vi "GEOM_GetCmdLineArgs.vi"() -> (6 "det_database":path, 8 "port":u16=4080, 13 "exit":bool, 14 "fpa":string)   [LabVIEW 2016]
panel:
  out "error out":errorcluster
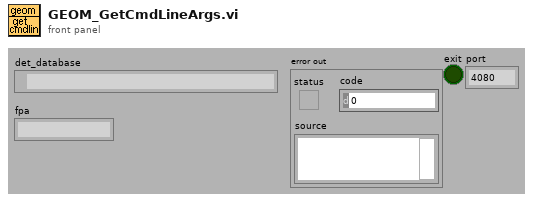
[diagram p1: front panel]
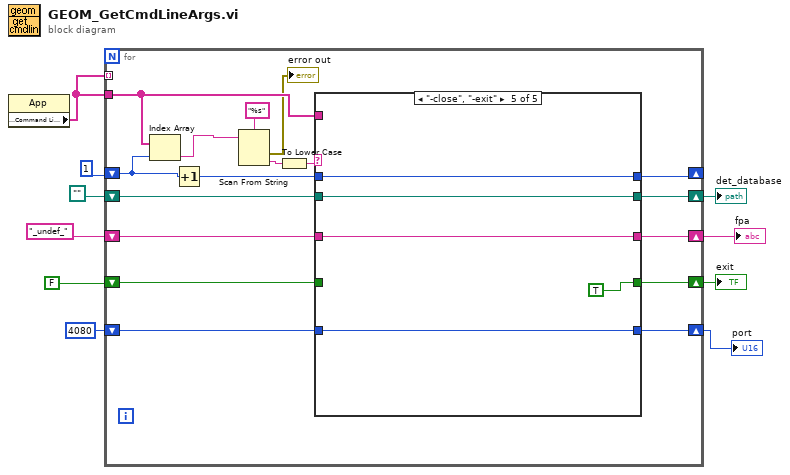
[diagram p0: block diagram]
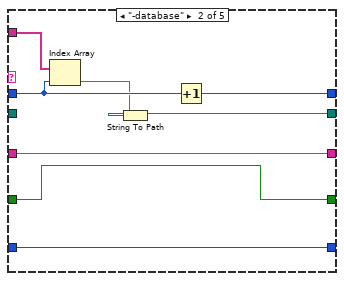
[diagram p3: hidden frame]
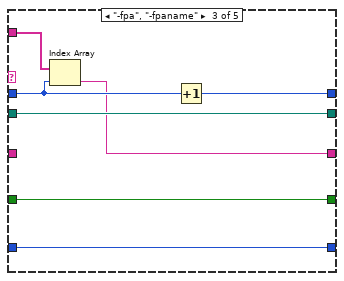
[diagram p4: hidden frame]
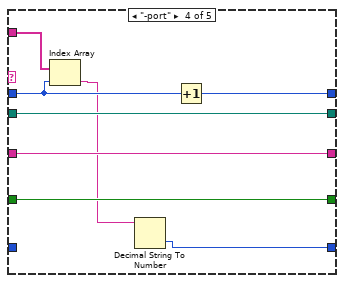
[diagram p5: hidden frame]
diagram:
  n1 = property class="App"() -> ("Application:Command Line Arguments"=w7:string[])  [unwired: 2 in, 2 out]
  n2 = for {
    shift-right: [w27] -> w9
    shift-left: path "" -> [w26]
    tunnel: w7 -> [w23]
    shift-right: [w21] -> _
    shift-left: 1 ("index") -> [w24]
    tunnel: w7 -> [_] mode=indexing
    shift-right: [w15] -> w6
    shift-left: "_undef_" ("element") -> [w16]
    shift-right: [w13] -> w3
    shift-left: FALSE -> [w14]
    shift-right: [w12] -> w2
    shift-left: 4080 -> [w11]
    n3 = Index Array(array=w23, index=w24) -> (element=w22:string)
    n4 = Increment(x=w24) -> (x+1=w25:i32)
    n5 = Scan From String(format string="%s", input string=w22) -> (error out=→"error out":errorcluster, output 1=w18:string)  [unwired: 2 in, 3 out]
    n6 = To Lower Case(string=w18) -> (all lower case string=w19:string)
    n7 = case shown="\"-close\", \"-exit\"" w19 {
      tunnel: [w32 w40 w44 w52 w59] -> w27
      tunnel: w26 -> [w32 _ w44 w52 w59]
      tunnel: w23 -> [_ w39 w47 w55 _]
      tunnel: w25 -> [w31 w38 w46 w54 w60]
      tunnel: [w31 w37 w45 w53 w60] -> w21
      tunnel: w16 -> [w30 w36 _ w50 w58]
      tunnel: [w30 w36 w43 w50 w58] -> w15
      tunnel: w14 -> [w29 w34 w42 w51 _]
      tunnel: [w29 w34 w42 w51 TRUE] -> w13
      tunnel: [w28 w33 w41 w48 w56] -> w12
      tunnel: w11 -> [w28 w33 w41 _ w56]
      frame Default {
      }
      frame "-database" {
        n8 = Index Array(array=w39, index=w38) -> (element=w35:string)
        n9 = String To Path(string=w35) -> (path=w40:path)
        n10 = Increment(x=w38) -> (x+1=w37:i32)
      }
      frame "-fpa", "-fpaname" {
        n11 = Index Array(array=w47, index=w46) -> (element=w43:string)
        n12 = Increment(x=w46) -> (x+1=w45:i32)
      }
      frame "-port" {
        n13 = Index Array(array=w55, index=w54) -> (element=w49:string)
        n14 = Decimal String To Number(string=w49) -> (number=w48:i32)  [unwired: 3 out]
        n15 = Increment(x=w54) -> (x+1=w53:i32)
      }
      frame "-close", "-exit" {
      }
    }
  }
  "det_database" <- w9
  "fpa" <- w6
  "exit" <- w3
  "port" <- w2
